vi "sub_GSlam_trans.vi"(11 "Direction Cosines 입력":dbl[][](array[numeric])) -> (3 "Direction Cosines 출력":dbl[][](array[numeric]))   [LabVIEW 2019]
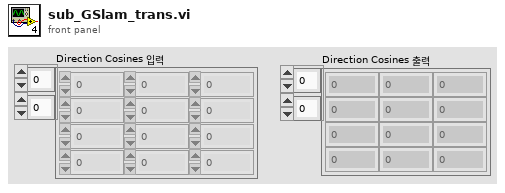
[diagram p1: front panel]
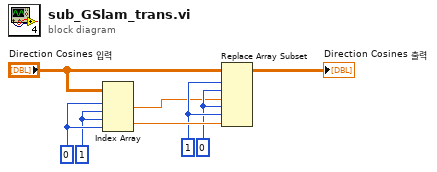
[diagram p0: block diagram]
diagram:
  w4 = 0 ("비활성화된 인덱스 (열)")
  w5 = 1 ("인덱스 (행)")
  w1 = 1 ("비활성화된 인덱스 (열)")
  w2 = 0 ("인덱스 (행)")
  n1 = Index Array(array="Direction Cosines 입력", index (row) #1=w2, index (col) #1=w1, index (row) #2=w1, index (col) #2=w2) -> (element #1=w3:dbl, element #2=w6:dbl)
  n2 = Replace Array Subset(array="Direction Cosines 입력", new element #1=w3, index (row) #1=w5, index (col) #1=w4, new element #2=w6, index (row) #2=w4, index (col) #2=w5) -> (→"Direction Cosines 출력":dbl[][])
